vi "DAQNavi Start Task.vi"(8 "error in (no error)":errorcluster, 11 "task in":i32) -> (0 "error out":errorcluster, 3 "task out":i32)   [LabVIEW 2020]
doc: "Transits the task to the running state to begin the measurement or generation. This VI is required for some applications and is optional for others."
uses:
  DAQNavi_LV.dll
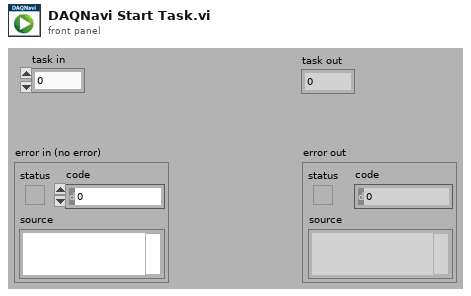
[diagram p1: front panel]
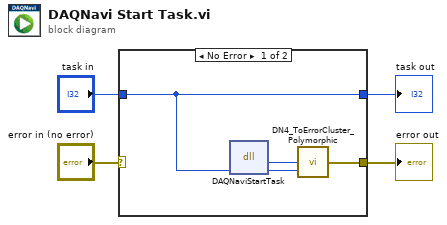
[diagram p0: block diagram]
diagram:
  n1 = case shown="No Error" "error in (no error)" {
    selector: "error in (no error)" -> [_ w10]
    tunnel: [w7 w10] -> w4
    tunnel: "task in" -> [w6 w9]
    tunnel: [w6 w9] -> w1
    frame No Error {
      n2 = dll-call lib="DAQNavi_LV.dll" fn="DAQNaviStartTask"("taskID"=w6) -> ("return type"=w8:i32, "taskID"=w5:i32)  [unwired: 3 in, 2 out]
      n3 = call "DN4_ToErrorCluster_Polymorphic.vi"("task id"=w5, "error code"=w8) -> ("error out"=w7:errorcluster)  [unwired: 3 out]
    }
    frame Error {
    }
  }
  "task out" <- w1
  "error out" <- w4
